vi "ep_Simulate Fluctuating Multiplier.vi"(0 "fluctuation level [%]":sgl=1.0) -> (4 "multiplier":sgl)   [LabVIEW 2011]
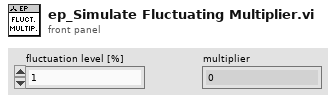
[diagram p1: front panel]
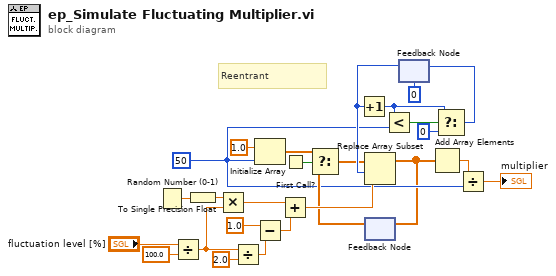
[diagram p0: block diagram]
diagram:
  w12 = 50 ("index")
  # "Reentrant"
  n1 = Random Number (0-1)() -> (number: 0 to 1=w21:dbl)
  n2 = Divide(x="fluctuation level [%]", y=sgl 100.0) -> (x/y=w3:sgl)
  n3 = To Single Precision Float(number=w21) -> (single precision float=w1:sgl)
  n4 = Multiply(x=w1, y=w3) -> (x*y=w22:sgl)
  n5 = Divide(x=w3, y=sgl 2.0) -> (x/y=w2:sgl)
  n6 = Initialize Array(sgl 1.0 ("element"), w12) -> (w10:sgl[])
  n7 = Subtract(x=sgl 1.0, y=w2) -> (x-y=w4:sgl)
  n8 = Add(x=w22, y=w4) -> (x+y=w26:sgl)
  n9 = First Call?() -> (First Call?: T/F=w19:bool)
  n10 = feedback #1() -> (w18:sgl[])  [unwired: 1 in]
  n11 = Select(t=w10, s=w19, f=w18) -> (s? t:f=w9:sgl[])
  n12 = feedback #2(0 ("index")) -> (w16:i32)
  n13 = Increment(x=w16) -> (x+1=w13:i32)
  n14 = Replace Array Subset(array=w9, new element=w26, index=w16) -> (w8:sgl[])
  n15 = feedback-in #1(w8) -> ()
  n16 = Less?(x=w13, y=w12) -> (x < y?=w15:bool)
  n17 = Add Array Elements(numeric array=w8) -> (sum=w17:sgl)
  n18 = Select(t=w13, s=w15, f=0) -> (s? t:f=w11:i32)
  n19 = feedback-in #2(w11) -> ()
  n20 = Divide(x=w17, y=w12) -> (x/y=→"multiplier":sgl)
